vi "Read WSserver Enqueuer.vi"(11 "WS Client in":refnum<class "WS Client.lvclass">) -> (2 "Stream Mediator.lvlib:Message Transport Queue.lvclass":refnum<class "Message Transport Queue.lvclass">, 3 "WS Client out":refnum<class "WS Client.lvclass">)   [LabVIEW 2016, in "WebSocket Networking.lvlib" / "WS Client.lvclass"]
uses:
  <userlib>/Common Components/WebSocket Networking/WS Client/WS Client.lvclass
  <userlib>/Composed Systems/Stream/Mediator/Classes/Message Transport Queue/Message Transport Queue.lvclass
  <userlib>/Common Components/WebSocket Networking/WS Client/WS Client.lvclass/WS Client.ctl
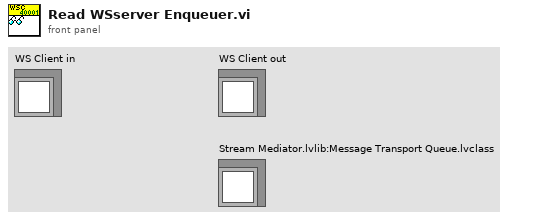
[diagram p1: front panel]
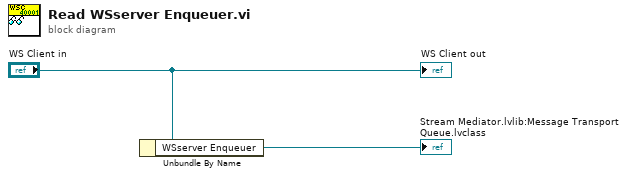
[diagram p0: block diagram]
diagram:
  n1 = Unbundle By Name("WS Client in") -> ("WSserver Enqueuer"=→"Stream Mediator.lvlib:Message Transport Queue.lvclass":refnum<class "Message Transport Queue.lvclass">)
  "WS Client out" <- "WS Client in"
